vi "Demo - Output PWM Signal and Read it Back with a Digital Input.vi"() -> ()   [LabVIEW 2021]
panel:
  out "Waveform Chart":i16(graph)
  in  "stop":bool
  in  "DAQ Address (IP or COM)":string="192.168.1.1"
  # "Instuctions for use:\nConnect a wire from DIO 0 to DIO 1, this\nallows the PWM signal to be output from\nchannel 0 and read back by channel 1."
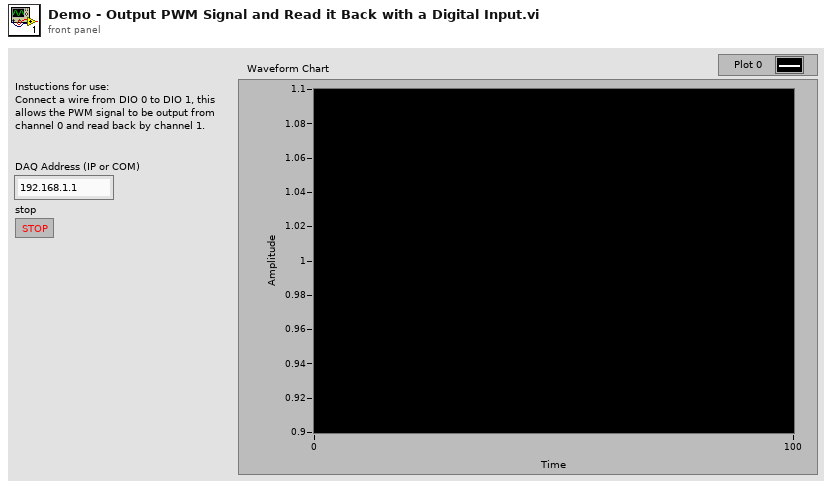
[diagram p1: front panel]
types:
  T1 = typedef "TypeDef - Cluster of DAQiFi Device Properties.ctl" = cluster{"IP Address":string, "MAC Address":string, "Serial Number":string, "Connection Type":T2, "Connected":bool, "TCP Network Connection":refnum<k5>, "USB Serial Connection":refnum<visa-resource-name>}
  T2 = typedef "Enum - Connection Type.ctl" = enum16{"USB", "TCP"}
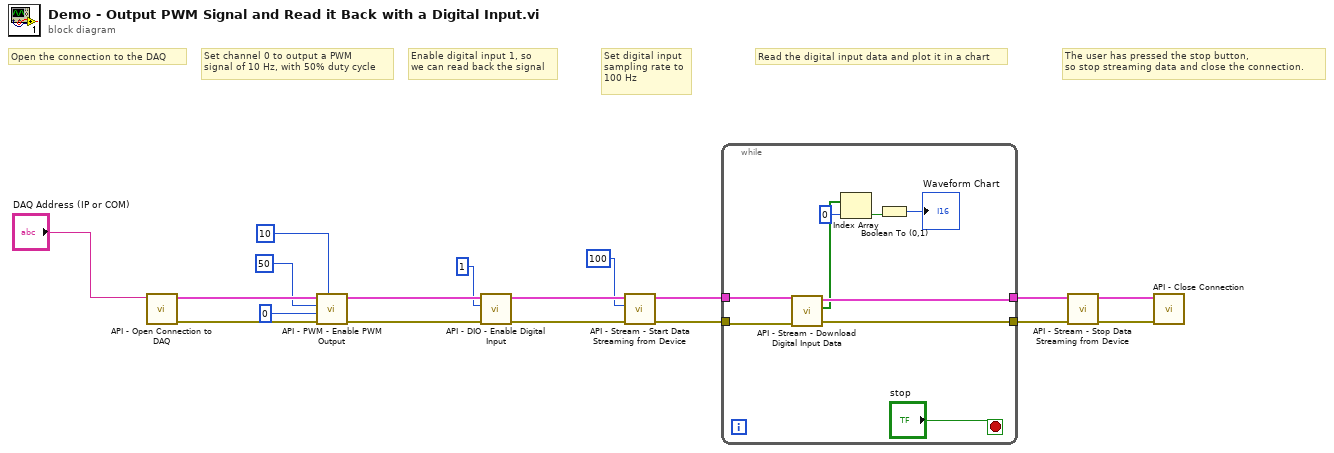
[diagram p0: block diagram]
diagram:
  # "The user has pressed the stop button,\nso stop streaming data and close the connection."
  # "Read the digital input data and plot it in a chart"
  # "Set digital input\nsampling rate to\n100 Hz"
  # "Enable digital input 1, so\nwe can read back the signal"
  # "Set channel 0 to output a PWM\nsignal of 10 Hz, with 50% duty cycle"
  # "Open the connection to the DAQ"
  n1 = call "API - Open Connection to DAQ.vi"("DAQ Address (IP or COM)"="DAQ Address (IP or COM)") -> ("error out"=w16:errorcluster, "DAQiFi Device Properties"=w17:T1)  [unwired: 9 in]
  n2 = call "API - PWM - Enable PWM Output.vi"("Frequency"=10, "error in"=w16, "PWM Channel Number"=0, "Duty Cycle (%)"=50, "DAQiFi Device Properties In"=w17) -> ("error out"=w11:errorcluster, "DAQiFi Device Properties Out"=w12:T1)  [unwired: 5 in]
  n3 = call "API - DIO - Enable Digital Input.vi"("error in"=w11, "Channel Number"=1, "DAQiFi Device Properties In"=w12) -> ("error out"=w7:errorcluster, "DAQiFi Device Properties Out"=w9:T1)  [unwired: 7 in]
  n4 = call "API - Stream - Start Data Streaming from Device.vi"("error in"=w7, "Streaming Rate (Hz)"=100, "DAQiFi Device Properties In"=w9) -> ("error out"=w6:errorcluster, "DAQiFi Device Properties Out"=w8:T1)  [unwired: 7 in]
  n5 = while {
    tunnel: [w24] -> w3
    tunnel: [w25] -> w4
    tunnel: w8 -> [w26]
    tunnel: w6 -> [w23]
    stop <- "stop" stop-if-true
    n6 = call "API - Stream - Download Digital Input Data.vi"("error in"=w23, "DAQiFi Device Properties In"=w26) -> ("error out"=w24:errorcluster, "Digital Inputs"=w22:bool[], "DAQiFi Device Properties Out"=w25:T1)  [unwired: 7 in]
    n7 = Index Array(array=w22, index=0) -> (element=w20:bool)
    n8 = Boolean To (0,1)(Boolean=w20) -> (0, 1=→"Waveform Chart":i16)
  }
  n9 = call "API - Stream - Stop Data Streaming from Device.vi"("error in"=w3, "DAQiFi Device Properties In"=w4) -> ("error out"=w2:errorcluster, "DAQiFi Device Properties Out"=w1:T1)  [unwired: 8 in]
  n10 = call "API - Close Connection.vi"("error in"=w2, "DAQiFi Device Properties In"=w1) -> ()  [unwired: 8 in, 2 out]
